vi "Set cif_manager_ClockStatus.vi"(7 "Complete Call (T)":bool=TRUE, 8 "error in (no error)":errorcluster, 10 "package_templatemessage":T1, 11 "gRPCid":T4) -> (0 "error out":errorcluster)   [LabVIEW 2021, in "CIF_Launcher_server.lvlib"]
uses:
  CIF_Launcher_server.lvlib
  <vilib>/gRPC/LabVIEW gRPC Library/Shared/grpcId.ctl
  cif_manager_ClockStatus.ctl
  cif_manager_ClockConversion.ctl
  cif_manager_TimePair.ctl
  cif_manager_ClockStatus_Flat.ctl
  cif_manager_ClockConversion_Flat.ctl
  cif_manager_TimePair_Flat.ctl
  dcc74a39-081a-4bdd-860b-8ed792803c96.vi
  RichToFlatcif_manager_ClockConversion.vi
  <vilib>/gRPC/LabVIEW gRPC Library/Shared/TranslateGrpcError.vi
  RichToFlatcif_manager_TimePair.vi
  <vilib>/gRPC/LabVIEW gRPC Library/Server API/Server/Get Server DLL Path.vi
  <vilib>/Utility/error.llb/Error Cluster From Error Code.vi
  <vilib>/gRPC/LabVIEW gRPC Library/grpc-lvsupport-release.lvlib
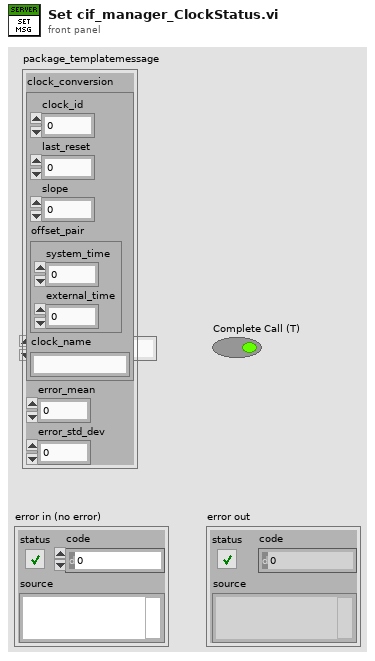
[diagram p1: front panel]
types:
  T1 = typedef "CIF_Launcher_server.lvlib/cif_manager_ClockStatus.ctl" = cluster{"clock_conversion":T2, "error_mean":i64, "error_std_dev":i64}
  T2 = typedef "CIF_Launcher_server.lvlib/cif_manager_ClockConversion.ctl" = cluster{"clock_id":u32, "last_reset":i64, "slope":dbl, "offset_pair":T3, "clock_name":string}
  T3 = typedef "CIF_Launcher_server.lvlib/cif_manager_TimePair.ctl" = cluster{"system_time":i64, "external_time":i64}
  T4 = typedef "grpc-lvsupport-release.lvlib/grpcId.ctl" = u64
  T5 = typedef "CIF_Launcher_server.lvlib/cif_manager_ClockStatus_Flat.ctl" = cluster{"clock_conversion":T6, "error_mean":i64, "error_std_dev":i64}
  T6 = typedef "CIF_Launcher_server.lvlib/cif_manager_ClockConversion_Flat.ctl" = cluster{"clock_id":u32, "last_reset":i64, "slope":dbl, "offset_pair":T7, "clock_name":string}
  T7 = typedef "CIF_Launcher_server.lvlib/cif_manager_TimePair_Flat.ctl" = cluster{"system_time":i64, "external_time":i64}
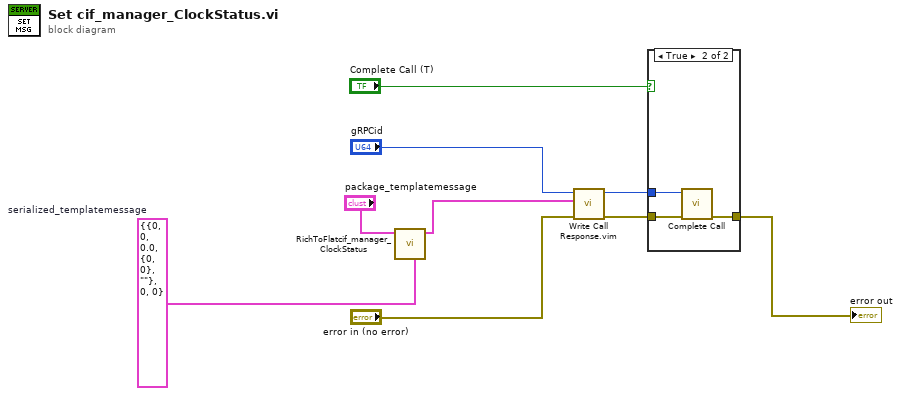
[diagram p0: block diagram]
diagram:
  w2 = T5 {"clock_conversion"={"clock_id"=0, "last_reset"=0, "slope"=0.0, "offset_pair"={"system_time"=0, "external_time"=0}, "clock_name"=""}, "error_mean"=0, "error_std_dev"=0}  # serialized_templatemessage
  n1 = call "RichToFlatcif_manager_ClockStatus.vi"("OutputClusterType"=w2, "InputCluster"="package_templatemessage") -> ("OutputCluster"=w1:T5)  [unwired: 9 in]
  n2 = call "Write Call Response.vim"("error in"="error in (no error)", "Response Data"=w1, "gRPCid in"="gRPCid") -> ("error out"=w6:errorcluster, "gRPCid out"=w7:T4)  [unwired: 7 in]
  n3 = case shown="True" "Complete Call (T)" {
    tunnel: [w10 w13] -> w9
    tunnel: w7 -> [_ w12]
    tunnel: w6 -> [w10 w11]
    frame False {
    }
    frame True {
      n4 = call <vilib>:"Complete Call.vi"("gRPCid"=w12, "error in"=w11) -> ("error out"=w13:errorcluster)  [unwired: 8 in]
    }
  }
  "error out" <- w9
